vi "W7X2DPut.vi"(4 "dimensions":i64[](array[numeric])=[1399090569999999999, -1], 6 "pulse_length":dbl, 7 "Unit":string, 8 "sample period":dbl, 9 "sample rate":u16, 10 "SigJSONbuffer":string, 11 "SigLabel":string) -> (0 "Parlog error out":errorcluster)   [LabVIEW 2014]
uses:
  <vilib>/httpClient/POSTBuffer.vi
  <vilib>/httpClient/LabVIEWHTTPClient.lvlib
panel:
  in  "values 2":T1(array[cluster])=[{"chanDescs"=[{"name"="E_Chan_1", "active"=1, "physicalQuantity"={"type"="A"}}, {"name"="E_Chan_2", "active"=1, "physicalQuantity"={"type"="A"}}, {"name"="E_Chan_3", "active"=1, "physicalQuantity"={"type"="A"}}, {"name"="E_Chan_4", "active"=1, "physicalQuantity"={"type"="A"}}, {"name"="E_Chan_5", "active"=1, "physicalQuantity"={"type"="A"}}, {"name"="E_Chan_6", "active"=1, "physicalQuantity"={"type"="A"}}, {"name"="E_Chan_7", "active"=1, "physicalQuantity"={"type"="A"}}, {"name"="E_Chan_8", "active"=1, "physicalQuantity"={"type"="A"}}, {"name"="E_Chan_9", "active"=1, "physicalQuantity"={"type"="A"}}, {"name"="E_Chan_10", "active"=1, "physicalQuantity"={"type"="A"}}, {"name"="E_Chan_11", "active"=1, "physicalQuantity"={"type"="A"}}, {"name"="E_Chan_12", "active"=1, "physicalQuantity"={"type"="A"}}, {"name"="E_Chan_13", "active"=1, "physicalQuantity"={"type"="A"}}, {"name"="E_Chan_14", "active"=1, "physicalQuantity"={"type"="A"}}, {"name"="E_Chan_15", "active"=1, "physicalQuantity"={"type"="A"}}, {"name"="E_Chan_16", "active"=1, "physicalQuantity"={"type"="A"}}, {"name"="E_Chan_17", "active"=1, "physicalQuantity"={"type"="A"}}, {"name"="E_Chan_18", "active"=1, "physicalQuantity"={"type"="A"}}, {"name"="E_Chan_19", "active"=1, "physicalQuantity"={"type"="A"}}, {"name"="E_Chan_20", "active"=1, "physicalQuantity"={"type"="A"}}, {"name"="E_Chan_21", "active"=1, "physicalQuantity"={"type"="A"}}, {"name"="E_Chan_22", "active"=1, "physicalQuantity"={"type"="A"}}, {"name"="E_Chan_23", "active"=1, "physicalQuantity"={"type"="A"}}, {"name"="E_Chan_24", "active"=1, "physicalQuantity"={"type"="A"}}, {"name"="E_Chan_25", "active"=1, "physicalQuantity"={"type"="A"}}, {"name"="E_Chan_26", "active"=1, "physicalQuantity"={"type"="A"}}, {"name"="E_Chan_27", "active"=1, "physicalQuantity"={"type"="A"}}, {"name"="E_Chan_28", "active"=1, "physicalQuantity"={"type"="A"}}, {"name"="E_Chan_29", "active"=1, "physicalQuantity"={"type"="A"}}, {"name"="E_Chan_30", "active"=1, "physicalQuantity"={"type"="A"}}, {"name"="E_Chan_31", "active"=1, "physicalQuantity"={"type"="A"}}, {"name"="E_Chan_32", "active"=1, "physicalQuantity"={"type"="A"}}, {"name"="E_Chan_33", "active"=1, "physicalQuantity"={"type"="A"}}, {"name"="E_Chan_34", "active"=1, "physicalQuantity"={"type"="A"}}, {"name"="E_Chan_35", "active"=1, "physicalQuantity"={"type"="A"}}, {"name"="E_Chan_36", "active"=1, "physicalQuantity"={"type"="A"}}, {"name"="E_Chan_37", "active"=1, "physicalQuantity"={"type"="A"}}, {"name"="E_Chan_38", "active"=1, "physicalQuantity"={"type"="A"}}, {"name"="E_Chan_39", "active"=1, "physicalQuantity"={"type"="A"}}, {"name"="E_Chan_40", "active"=1, "physicalQuantity"={"type"="A"}}, {"name"="E_Chan_41", "active"=1, "physicalQuantity"={"type"="A"}}, {"name"="E_Chan_42", "active"=1, "physicalQuantity"={"type"="A"}}, {"name"="E_Chan_43", "active"=1, "physicalQuantity"={"type"="A"}}, {"name"="E_Chan_44", "active"=1, "physicalQuantity"={"type"="A"}}, {"name"="E_Chan_45", "active"=1, "physicalQuantity"={"type"="A"}}, {"name"="E_Chan_46", "active"=1, "physicalQuantity"={"type"="A"}}, {"name"="E_Chan_47", "active"=1, "physicalQuantity"={"type"="A"}}, {"name"="E_Chan_48", "active"=1, "physicalQuantity"={"type"="A"}}, {"name"="E_Chan_49", "active"=1, "physicalQuantity"={"type"="A"}}, {"name"="E_Chan_50", "active"=1, "physicalQuantity"={"type"="A"}}, {"name"="E_Chan_51", "active"=1, "physicalQuantity"={"type"="A"}}, {"name"="E_Chan_52", "active"=1, "physicalQuantity"={"type"="A"}}, {"name"="E_Chan_53", "active"=1, "physicalQuantity"={"type"="A"}}, {"name"="E_Chan_54", "active"=1, "physicalQuantity"={"type"="A"}}, {"name"="E_Chan_55", "active"=1, "physicalQuantity"={"type"="A"}}, {"name"="E_Chan_56", "active"=1, "physicalQuantity"={"type"="A"}}, {"name"="E_Chan_57", "active"=1, "physicalQuantity"={"type"="A"}}, {"name"="E_Chan_58", "active"=1, "physicalQuantity"={"type"="A"}}, {"name"="E_Chan_59", "active"=1, "physicalQuantity"={"type"="A"}}, {"name"="E_Chan_60", "active"=1, "physicalQuantity"={"type"="A"}}, {"name"="E_Chan_61", "active"=1, "physicalQuantity"={"type"="A"}}, {"name"="E_Chan_62", "active"=1, "physicalQuantity"={"type"="A"}}, {"name"="E_Chan_63", "active"=1, "physicalQuantity"={"type"="A"}}, {"name"="E_Chan_64", "active"=1, "physicalQuantity"={"type"="A"}}, {"name"="E_Chan_65", "active"=1, "physicalQuantity"={"type"="A"}}, {"name"="E_Chan_66", "active"=1, "physicalQuantity"={"type"="A"}}, {"name"="E_Chan_67", "active"=1, "physicalQuantity"={"type"="A"}}, {"name"="E_Chan_68", "active"=1, "physicalQuantity"={"type"="A"}}, {"name"="E_Chan_69", "active"=1, "physicalQuantity"={"type"="A"}}, {"name"="E_Chan_70", "active"=1, "physicalQuantity"={"type"="A"}}, {"name"="E_Chan_71", "active"=1, "physicalQuantity"={"type"="A"}}, {"name"="E_Chan_72", "active"=1, "physicalQuantity"={"type"="A"}}, {"name"="E_Chan_73", "active"=1, "physicalQuantity"={"type"="A"}}, {"name"="E_Chan_74", "active"=1, "physicalQuantity"={"type"="A"}}, {"name"="E_Chan_75", "active"=1, "physicalQuantity"={"type"="A"}}, {"name"="E_Chan_76", "active"=1, "physicalQuantity"={"type"="A"}}, {"name"="E_Chan_77", "active"=1, "physicalQuantity"={"type"="A"}}, {"name"="E_Chan_78", "active"=1, "physicalQuantity"={"type"="A"}}, {"name"="E_Chan_79", "active"=1, "physicalQuantity"={"type"="A"}}, {"name"="E_Chan_80", "active"=1, "physicalQuantity"={"type"="A"}}, {"name"="E_Chan_81", "active"=1, "physicalQuantity"={"type"="A"}}, {"name"="E_Chan_82", "active"=1, "physicalQuantity"={"type"="A"}}, {"name"="E_Chan_83", "active"=1, "physicalQuantity"={"type"="A"}}, {"name"="E_Chan_84", "active"=1, "physicalQuantity"={"type"="A"}}, {"name"="E_Chan_85", "active"=1, "physicalQuantity"={"type"="A"}}, {"name"="E_Chan_86", "active"=1, "physicalQuantity"={"type"="A"}}, {"name"="E_Chan_87", "active"=1, "physicalQuantity"={"type"="A"}}, {"name"="E_Chan_88", "active"=1, "physicalQuantity"={"type"="A"}}, {"name"="E_Chan_89", "active"=1, "physicalQuantity"={"type"="A"}}, {"name"="E_Chan_90", "active"=1, "physicalQuantity"={"type"="A"}}, {"name"="E_Chan_91", "active"=1, "physicalQuantity"={"type"="A"}}, {"name"="E_Chan_92", "active"=1, "physicalQuantity"={"type"="A"}}, {"name"="E_Chan_93", "active"=1, "physicalQuantity"={"type"="A"}}, {"name"="E_Chan_94", "active"=1, "physicalQuantity"={"type"="A"}}, {"name"="E_Chan_95", "active"=1, "physicalQuantity"={"type"="A"}}, {"name"="E_Chan_96", "active"=1, "physicalQuantity"={"type"="A"}}, {"name"="E_Chan_97", "active"=1, "physicalQuantity"={"type"="A"}}, {"name"="E_Chan_98", "active"=1, "physicalQuantity"={"type"="A"}}, {"name"="E_Chan_99", "active"=1, "physicalQuantity"={"type"="A"}}, {"name"="E_Chan_100", "active"=1, "physicalQuantity"={"type"="A"}}, {"name"="E_Chan_101", "active"=1, "physicalQuantity"={"type"="A"}}, {"name"="E_Chan_102", "active"=1, "physicalQuantity"={"type"="A"}}, {"name"="E_Chan_103", "active"=1, "physicalQuantity"={"type"="A"}}, {"name"="E_Chan_104", "active"=1, "physicalQuantity"={"type"="A"}}, {"name"="E_Chan_105", "active"=1, "physicalQuantity"={"type"="A"}}, {"name"="E_Chan_106", "active"=1, "physicalQuantity"={"type"="A"}}, {"name"="E_Chan_107", "active"=1, "physicalQuantity"={"type"="A"}}, {"name"="E_Chan_108", "active"=1, "physicalQuantity"={"type"="A"}}, {"name"="E_Chan_109", "active"=1, "physicalQuantity"={"type"="A"}}, {"name"="E_Chan_110", "active"=1, "physicalQuantity"={"type"="A"}}, {"name"="E_Chan_111", "active"=1, "physicalQuantity"={"type"="A"}}, {"name"="E_Chan_112", "active"=1, "physicalQuantity"={"type"="A"}}, {"name"="E_Chan_113", "active"=1, "physicalQuantity"={"type"="A"}}, {"name"="E_Chan_114", "active"=1, "physicalQuantity"={"type"="A"}}, {"name"="E_Chan_115", "active"=1, "physicalQuantity"={"type"="A"}}, {"name"="E_Chan_116", "active"=1, "physicalQuantity"={"type"="A"}}, {"name"="E_Chan_117", "active"=1, "physicalQuantity"={"type"="A"}}, {"name"="E_Chan_118", "active"=1, "physicalQuantity"={"type"="A"}}, {"name"="E_Chan_119", "active"=1, "physicalQuantity"={"type"="A"}}, {"name"="E_Chan_120", "active"=1, "physicalQuantity"={"type"="A"}}, {"name"="E_Chan_121", "active"=1, "physicalQuantity"={"type"="A"}}, {"name"="E_Chan_122", "active"=1, "physicalQuantity"={"type"="A"}}, {"name"="E_Chan_123", "active"=1, "physicalQuantity"={"type"="A"}}, {"name"="E_Chan_124", "active"=1, "physicalQuantity"={"type"="A"}}, {"name"="E_Chan_125", "active"=1, "physicalQuantity"={"type"="A"}}, {"name"="E_Chan_126", "active"=1, "physicalQuantity"={"type"="A"}}, {"name"="E_Chan_127", "active"=1, "physicalQuantity"={"type"="A"}}, {"name"="E_Chan_128", "active"=1, "physicalQuantity"={"type"="A"}}], "detector"="Au_Kapton", "NChannels"=128, "ADCBits"=16, "CalStep1 (V)"="2.5", "CalStep2 (V)"="3.7"}]
  out "JSON string":string
  in  "values":T2(array[cluster])=[{"sample_period"=0.004, "sample_rate"=2500, "pulse_length"=4.0, "detector"="Au_Kapton", "NChannels"=128, "ADCBits"=16, "BridgeVoltage (V)"=5.0, "chanDescs"=[{"name"="E_Chan_1", "active"=1, "physicalQuantity"={"type"="A"}}, {"name"="E_Chan_2", "active"=1, "physicalQuantity"={"type"="A"}}, {"name"="E_Chan_3", "active"=1, "physicalQuantity"={"type"="A"}}, {"name"="E_Chan_4", "active"=1, "physicalQuantity"={"type"="A"}}, {"name"="E_Chan_5", "active"=1, "physicalQuantity"={"type"="A"}}, {"name"="E_Chan_6", "active"=1, "physicalQuantity"={"type"="A"}}, {"name"="E_Chan_7", "active"=1, "physicalQuantity"={"type"="A"}}, {"name"="E_Chan_8", "active"=1, "physicalQuantity"={"type"="A"}}, {"name"="E_Chan_9", "active"=1, "physicalQuantity"={"type"="A"}}, {"name"="E_Chan_10", "active"=1, "physicalQuantity"={"type"="A"}}, {"name"="E_Chan_11", "active"=1, "physicalQuantity"={"type"="A"}}, {"name"="E_Chan_12", "active"=1, "physicalQuantity"={"type"="A"}}, {"name"="E_Chan_13", "active"=1, "physicalQuantity"={"type"="A"}}, {"name"="E_Chan_14", "active"=1, "physicalQuantity"={"type"="A"}}, {"name"="E_Chan_15", "active"=1, "physicalQuantity"={"type"="A"}}, {"name"="E_Chan_16", "active"=1, "physicalQuantity"={"type"="A"}}, {"name"="E_Chan_17", "active"=1, "physicalQuantity"={"type"="A"}}, {"name"="E_Chan_18", "active"=1, "physicalQuantity"={"type"="A"}}, {"name"="E_Chan_19", "active"=1, "physicalQuantity"={"type"="A"}}, {"name"="E_Chan_20", "active"=1, "physicalQuantity"={"type"="A"}}, {"name"="E_Chan_21", "active"=1, "physicalQuantity"={"type"="A"}}, {"name"="E_Chan_22", "active"=1, "physicalQuantity"={"type"="A"}}, {"name"="E_Chan_23", "active"=1, "physicalQuantity"={"type"="A"}}, {"name"="E_Chan_24", "active"=1, "physicalQuantity"={"type"="A"}}, {"name"="E_Chan_25", "active"=1, "physicalQuantity"={"type"="A"}}, {"name"="E_Chan_26", "active"=1, "physicalQuantity"={"type"="A"}}, {"name"="E_Chan_27", "active"=1, "physicalQuantity"={"type"="A"}}, {"name"="E_Chan_28", "active"=1, "physicalQuantity"={"type"="A"}}, {"name"="E_Chan_29", "active"=1, "physicalQuantity"={"type"="A"}}, {"name"="E_Chan_30", "active"=1, "physicalQuantity"={"type"="A"}}, {"name"="E_Chan_31", "active"=1, "physicalQuantity"={"type"="A"}}, {"name"="E_Chan_32", "active"=1, "physicalQuantity"={"type"="A"}}, {"name"="E_Chan_33", "active"=1, "physicalQuantity"={"type"="A"}}, {"name"="E_Chan_34", "active"=1, "physicalQuantity"={"type"="A"}}, {"name"="E_Chan_35", "active"=1, "physicalQuantity"={"type"="A"}}, {"name"="E_Chan_36", "active"=1, "physicalQuantity"={"type"="A"}}, {"name"="E_Chan_37", "active"=1, "physicalQuantity"={"type"="A"}}, {"name"="E_Chan_38", "active"=1, "physicalQuantity"={"type"="A"}}, {"name"="E_Chan_39", "active"=1, "physicalQuantity"={"type"="A"}}, {"name"="E_Chan_40", "active"=1, "physicalQuantity"={"type"="A"}}, {"name"="E_Chan_41", "active"=1, "physicalQuantity"={"type"="A"}}, {"name"="E_Chan_42", "active"=1, "physicalQuantity"={"type"="A"}}, {"name"="E_Chan_43", "active"=1, "physicalQuantity"={"type"="A"}}, {"name"="E_Chan_44", "active"=1, "physicalQuantity"={"type"="A"}}, {"name"="E_Chan_45", "active"=1, "physicalQuantity"={"type"="A"}}, {"name"="E_Chan_46", "active"=1, "physicalQuantity"={"type"="A"}}, {"name"="E_Chan_47", "active"=1, "physicalQuantity"={"type"="A"}}, {"name"="E_Chan_48", "active"=1, "physicalQuantity"={"type"="A"}}, {"name"="E_Chan_49", "active"=1, "physicalQuantity"={"type"="A"}}, {"name"="E_Chan_50", "active"=1, "physicalQuantity"={"type"="A"}}, {"name"="E_Chan_51", "active"=1, "physicalQuantity"={"type"="A"}}, {"name"="E_Chan_52", "active"=1, "physicalQuantity"={"type"="A"}}, {"name"="E_Chan_53", "active"=1, "physicalQuantity"={"type"="A"}}, {"name"="E_Chan_54", "active"=1, "physicalQuantity"={"type"="A"}}, {"name"="E_Chan_55", "active"=1, "physicalQuantity"={"type"="A"}}, {"name"="E_Chan_56", "active"=1, "physicalQuantity"={"type"="A"}}, {"name"="E_Chan_57", "active"=1, "physicalQuantity"={"type"="A"}}, {"name"="E_Chan_58", "active"=1, "physicalQuantity"={"type"="A"}}, {"name"="E_Chan_59", "active"=1, "physicalQuantity"={"type"="A"}}, {"name"="E_Chan_60", "active"=1, "physicalQuantity"={"type"="A"}}, {"name"="E_Chan_61", "active"=1, "physicalQuantity"={"type"="A"}}, {"name"="E_Chan_62", "active"=1, "physicalQuantity"={"type"="A"}}, {"name"="E_Chan_63", "active"=1, "physicalQuantity"={"type"="A"}}, {"name"="E_Chan_64", "active"=1, "physicalQuantity"={"type"="A"}}, {"name"="E_Chan_65", "active"=1, "physicalQuantity"={"type"="A"}}, {"name"="E_Chan_66", "active"=1, "physicalQuantity"={"type"="A"}}, {"name"="E_Chan_67", "active"=1, "physicalQuantity"={"type"="A"}}, {"name"="E_Chan_68", "active"=1, "physicalQuantity"={"type"="A"}}, {"name"="E_Chan_69", "active"=1, "physicalQuantity"={"type"="A"}}, {"name"="E_Chan_70", "active"=1, "physicalQuantity"={"type"="A"}}, {"name"="E_Chan_71", "active"=1, "physicalQuantity"={"type"="A"}}, {"name"="E_Chan_72", "active"=1, "physicalQuantity"={"type"="A"}}, {"name"="E_Chan_73", "active"=1, "physicalQuantity"={"type"="A"}}, {"name"="E_Chan_74", "active"=1, "physicalQuantity"={"type"="A"}}, {"name"="E_Chan_75", "active"=1, "physicalQuantity"={"type"="A"}}, {"name"="E_Chan_76", "active"=1, "physicalQuantity"={"type"="A"}}, {"name"="E_Chan_77", "active"=1, "physicalQuantity"={"type"="A"}}, {"name"="E_Chan_78", "active"=1, "physicalQuantity"={"type"="A"}}, {"name"="E_Chan_79", "active"=1, "physicalQuantity"={"type"="A"}}, {"name"="E_Chan_80", "active"=1, "physicalQuantity"={"type"="A"}}, {"name"="E_Chan_81", "active"=1, "physicalQuantity"={"type"="A"}}, {"name"="E_Chan_82", "active"=1, "physicalQuantity"={"type"="A"}}, {"name"="E_Chan_83", "active"=1, "physicalQuantity"={"type"="A"}}, {"name"="E_Chan_84", "active"=1, "physicalQuantity"={"type"="A"}}, {"name"="E_Chan_85", "active"=1, "physicalQuantity"={"type"="A"}}, {"name"="E_Chan_86", "active"=1, "physicalQuantity"={"type"="A"}}, {"name"="E_Chan_87", "active"=1, "physicalQuantity"={"type"="A"}}, {"name"="E_Chan_88", "active"=1, "physicalQuantity"={"type"="A"}}, {"name"="E_Chan_89", "active"=1, "physicalQuantity"={"type"="A"}}, {"name"="E_Chan_90", "active"=1, "physicalQuantity"={"type"="A"}}, {"name"="E_Chan_91", "active"=1, "physicalQuantity"={"type"="A"}}, {"name"="E_Chan_92", "active"=1, "physicalQuantity"={"type"="A"}}, {"name"="E_Chan_93", "active"=1, "physicalQuantity"={"type"="A"}}, {"name"="E_Chan_94", "active"=1, "physicalQuantity"={"type"="A"}}, {"name"="E_Chan_95", "active"=1, "physicalQuantity"={"type"="A"}}, {"name"="E_Chan_96", "active"=1, "physicalQuantity"={"type"="A"}}, {"name"="E_Chan_97", "active"=1, "physicalQuantity"={"type"="A"}}, {"name"="E_Chan_98", "active"=1, "physicalQuantity"={"type"="A"}}, {"name"="E_Chan_99", "active"=1, "physicalQuantity"={"type"="A"}}, {"name"="E_Chan_100", "active"=1, "physicalQuantity"={"type"="A"}}, {"name"="E_Chan_101", "active"=1, "physicalQuantity"={"type"="A"}}, {"name"="E_Chan_102", "active"=1, "physicalQuantity"={"type"="A"}}, {"name"="E_Chan_103", "active"=1, "physicalQuantity"={"type"="A"}}, {"name"="E_Chan_104", "active"=1, "physicalQuantity"={"type"="A"}}, {"name"="E_Chan_105", "active"=1, "physicalQuantity"={"type"="A"}}, {"name"="E_Chan_106", "active"=1, "physicalQuantity"={"type"="A"}}, {"name"="E_Chan_107", "active"=1, "physicalQuantity"={"type"="A"}}, {"name"="E_Chan_108", "active"=1, "physicalQuantity"={"type"="A"}}, {"name"="E_Chan_109", "active"=1, "physicalQuantity"={"type"="A"}}, {"name"="E_Chan_110", "active"=1, "physicalQuantity"={"type"="A"}}, {"name"="E_Chan_111", "active"=1, "physicalQuantity"={"type"="A"}}, {"name"="E_Chan_112", "active"=1, "physicalQuantity"={"type"="A"}}, {"name"="E_Chan_113", "active"=1, "physicalQuantity"={"type"="A"}}, {"name"="E_Chan_114", "active"=1, "physicalQuantity"={"type"="A"}}, {"name"="E_Chan_115", "active"=1, "physicalQuantity"={"type"="A"}}, {"name"="E_Chan_116", "active"=1, "physicalQuantity"={"type"="A"}}, {"name"="E_Chan_117", "active"=1, "physicalQuantity"={"type"="A"}}, {"name"="E_Chan_118", "active"=1, "physicalQuantity"={"type"="A"}}, {"name"="E_Chan_119", "active"=1, "physicalQuantity"={"type"="A"}}, {"name"="E_Chan_120", "active"=1, "physicalQuantity"={"type"="A"}}, {"name"="E_Chan_121", "active"=1, "physicalQuantity"={"type"="A"}}, {"name"="E_Chan_122", "active"=1, "physicalQuantity"={"type"="A"}}, {"name"="E_Chan_123", "active"=1, "physicalQuantity"={"type"="A"}}, {"name"="E_Chan_124", "active"=1, "physicalQuantity"={"type"="A"}}, {"name"="E_Chan_125", "active"=1, "physicalQuantity"={"type"="A"}}, {"name"="E_Chan_126", "active"=1, "physicalQuantity"={"type"="A"}}, {"name"="E_Chan_127", "active"=1, "physicalQuantity"={"type"="A"}}, {"name"="E_Chan_128", "active"=1, "physicalQuantity"={"type"="A"}}]}]
  out "body":string
  out "headers":string
  out "body Parlog":string
  out "headers parms":string
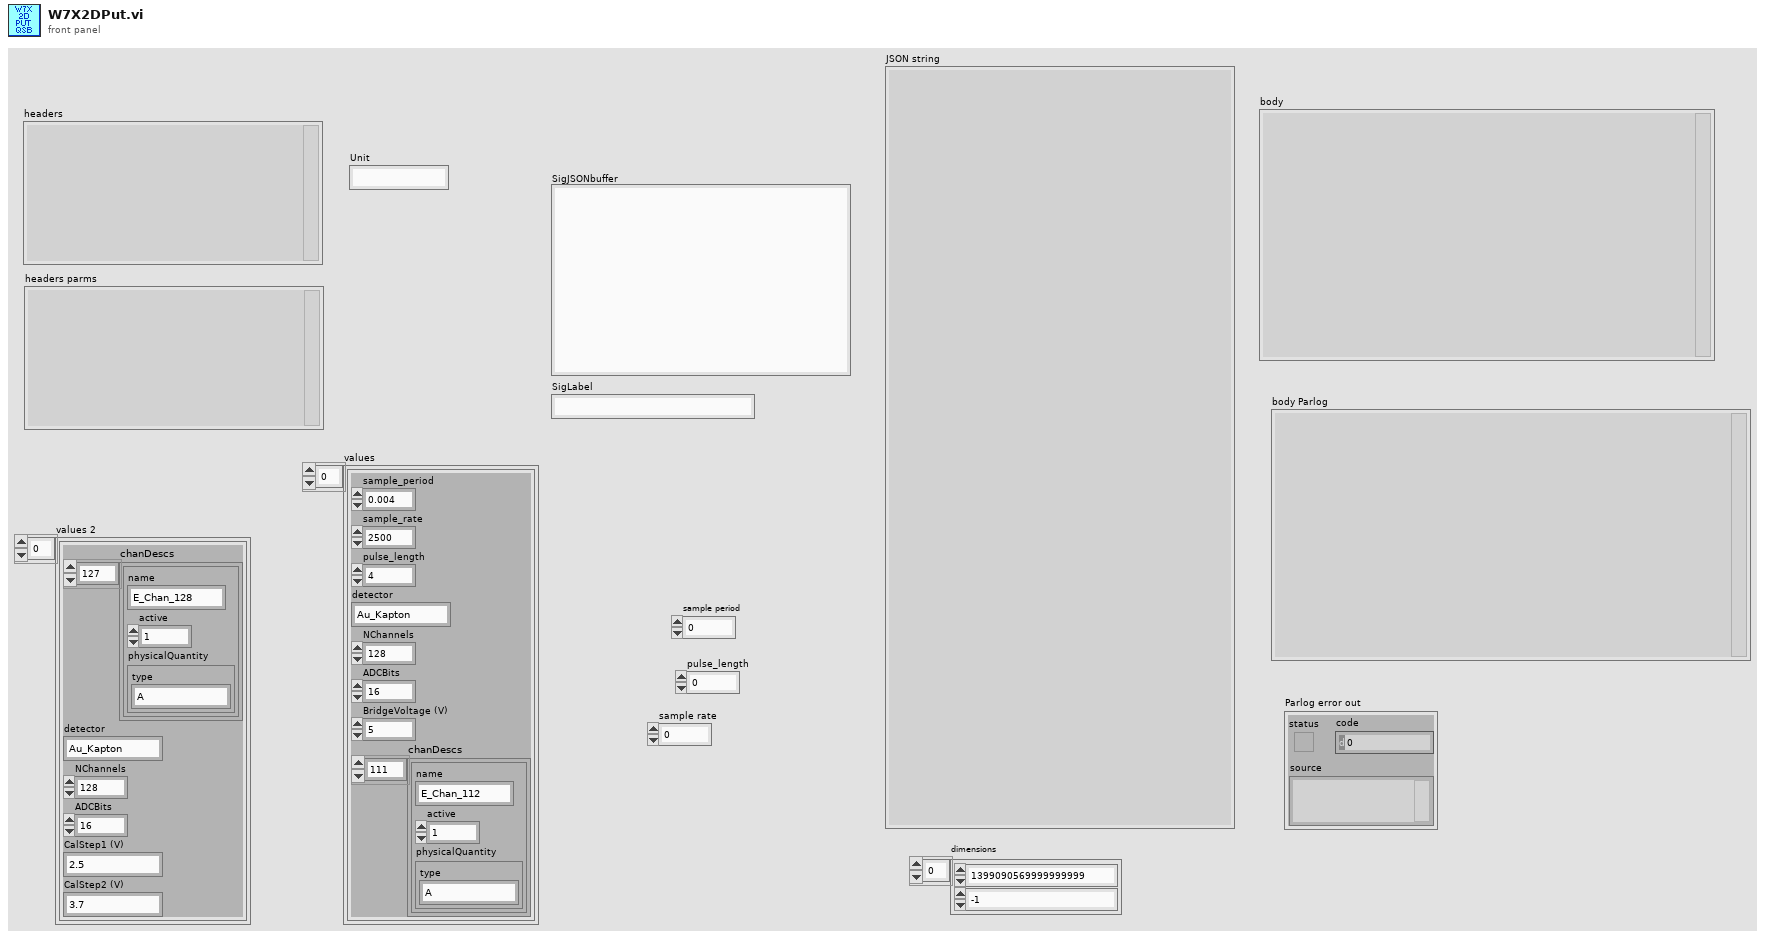
[diagram p1: front panel]
types:
  T1 = cluster{"chanDescs":cluster{"name":string, "active":i32, "physicalQuantity":cluster{"type":string}}[], "detector":string, "NChannels":u16, "ADCBits":u16, "CalStep1 (V)":string, "CalStep2 (V)":string}[]
  T2 = cluster{"sample_period":dbl, "sample_rate":u16, "pulse_length":dbl, "detector":string, "NChannels":u16, "ADCBits":u16, "BridgeVoltage (V)":sgl, "chanDescs":cluster{"name":string, "active":i32, "physicalQuantity":cluster{"type":string}}[]}[]
  T3 = cluster{"sample_period":dbl, "sample_rate":u16, "pulse_length":dbl, "detector":string, "NChannels":u16, "ADCBits":u16, "BridgeVoltage (V)":sgl, "chanDescs":cluster{"name":string, "active":i32, "physicalQuantity":cluster{"type":string}}[]}
  T4 = cluster{"name":string, "active":i32, "physicalQuantity":cluster{"type":string}}[]
  T5 = cluster{"name":string, "active":i32, "physicalQuantity":cluster{"type":string}}
  T6 = typedef "LabVIEWHTTPClient.lvlib/ClientHandle.ctl" = refnum<k1>
  T7 = cluster{"label":string, "values":cluster{"sample_period":dbl, "sample_rate":u16, "pulse_length":dbl, "detector":string, "NChannels":u16, "ADCBits":u16, "BridgeVoltage (V)":sgl, "chanDescs":cluster{"name":string, "active":i32, "physicalQuantity":cluster{"type":string}}[]}[], "dimensions":i64[]}
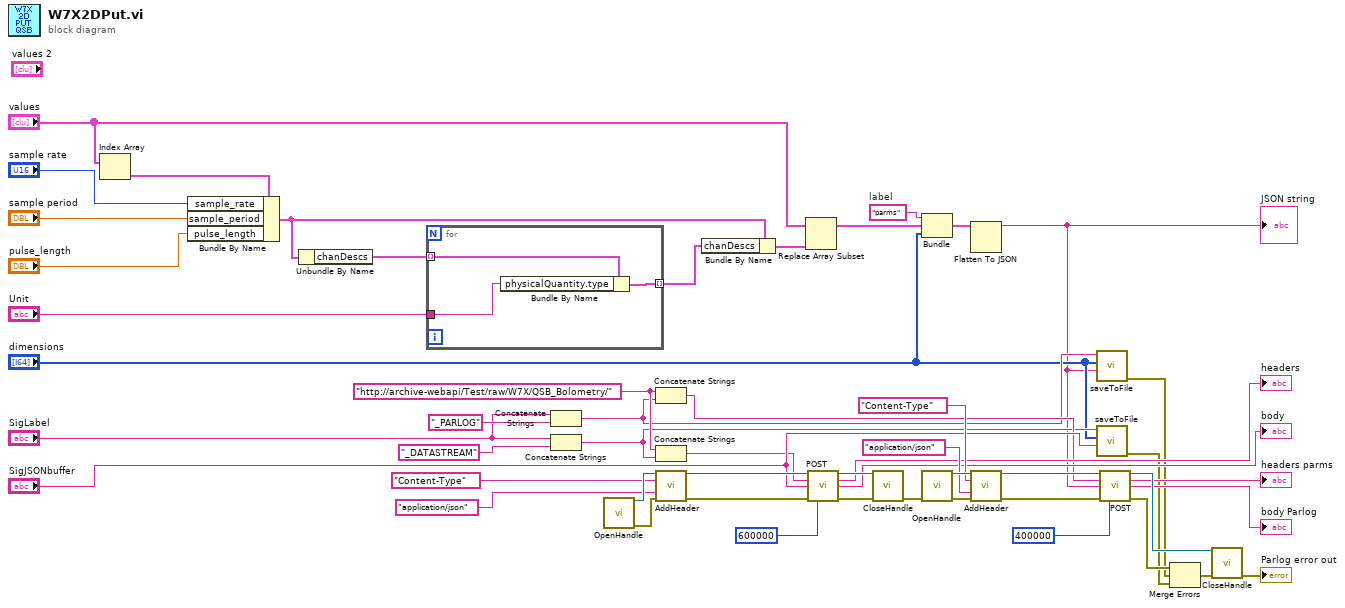
[diagram p0: block diagram]
diagram:
  w26 = "parms"  # label
  w9 = "http://archive-webapi/Test/raw/W7X/QSB_Bolometry/" ("url")
  n1 = Index Array(array="values") -> (element=w21:T3)  [unwired: 1 in]
  n2 = Bundle By Name(cluster=w21, "sample_rate"="sample rate", "sample_period"="sample period", "pulse_length"="pulse_length") -> (w17:T3)
  n3 = Unbundle By Name(w17) -> ("chanDescs"=w16:T4)
  n4 = for {
    tunnel: w16 -> [w54] mode=indexing
    tunnel: [w53] -> w15 mode=indexing
    tunnel: "Unit" -> [w52]
    n5 = Bundle By Name(cluster=w54, "physicalQuantity.type"=w52) -> (w53:T5)
  }
  n6 = Concatenate Strings("SigLabel", "_PARLOG" ("replace string (\"\")")) -> (w7:string)
  n7 = Concatenate Strings("SigLabel", "_DATASTREAM" ("string")) -> (w8:string)
  n8 = call <vilib>:"OpenHandle.vi"() -> ("client handle out"=w36:T6, "error out"=w35:errorcluster)  [unwired: 14 in]
  n9 = Concatenate Strings(w9, w7) -> (w10:string)
  n10 = Concatenate Strings(w9, w8) -> (w11:string)
  n11 = call <vilib>:"AddHeader.vi"("client handle"=w36, "header"="Content-Type", "value"="application/json", "error in (no error)"=w35) -> ("client handle out"=w34:T6, "error out"=w33:errorcluster)  [unwired: 10 in]
  n12 = Bundle By Name(cluster=w17, "chanDescs"=w15) -> (w19:T3)
  n13 = Replace Array Subset(array="values", new element=w19) -> (w18:T2)  [unwired: 1 in]
  n14 = call-poly <vilib>:"POST.vi"("client handle"=w34, "url"=w11, "buffer"="SigJSONbuffer", "error in (no error)"=w33, "timeout (10000)"=600000) -> ("client handle out"=w39:T6, "headers"=→"headers":string, "body"=→"body":string, "error out"=w38:errorcluster)  [unwired: 7 in]
  n15 = call <vilib>:"CloseHandle.vi"("client handle"=w39, "error in (no error)"=w38) -> ("error out"=w1:errorcluster)  [unwired: 13 in]
  n16 = Bundle("label"=w26, "values"=w18, "dimensions"="dimensions") -> (w25:T7)  [unwired: 1 in]
  n17 = call <vilib>:"OpenHandle.vi"("error in (no error)"=w1) -> ("client handle out"=w48:T6, "error out"=w47:errorcluster)  [unwired: 13 in]
  n18 = Flatten To JSON(anything=w25) -> (JSON string=w5:string)  [unwired: 2 in, 1 out]
  "JSON string" <- w5
  n19 = call <vilib>:"AddHeader.vi"("client handle"=w48, "header"="Content-Type", "value"="application/json", "error in (no error)"=w47) -> ("client handle out"=w46:T6, "error out"=w45:errorcluster)  [unwired: 10 in]
  n20 = call "saveToFile.vi"("SigJSONbuffer"=w5, "dimensions"="dimensions", "String"=w7) -> ("error out"=w3:errorcluster)  [unwired: 8 in]
  n21 = call "saveToFile.vi"("SigJSONbuffer"="SigJSONbuffer", "dimensions"="dimensions", "String"=w8) -> ("error out"=w2:errorcluster)  [unwired: 8 in]
  n22 = call-poly <vilib>:"POST.vi"("client handle"=w46, "url"=w10, "buffer"=w5, "error in (no error)"=w45, "timeout (10000)"=400000) -> ("client handle out"=w51:T6, "headers"=→"headers parms":string, "body"=→"body Parlog":string, "error out"=w50:errorcluster)  [unwired: 7 in]
  n23 = Merge Errors(w50, w3, w2) -> (w4:errorcluster)
  n24 = call <vilib>:"CloseHandle.vi"("client handle"=w51, "error in (no error)"=w4) -> ("error out"=→"Parlog error out":errorcluster)  [unwired: 13 in]
